vi "Struct PLC Byte Stream to G Object.vi"(8 "error in (no error)":errorcluster, 9 "[Sub-Item Type Information]":T1[](array[typedef]), 10 "Byte Stream":u8[](array[numeric]), 11 "TwinCAT ADS in":refnum<class "TwinCAT ADS.lvclass">) -> (0 "error out":errorcluster, 2 "Value":variant, 3 "TwinCAT ADS out":refnum<class "TwinCAT ADS.lvclass">)   [LabVIEW 2018, in "TwinCAT ADS.lvclass"]
uses:
  TwinCAT ADS.lvclass
  Controls/PLC Sub-Item Type Descriptor.ctl
  Controls/PLC Type.ctl
  Controls/PLC Array Type Descriptor.ctl
  Standard PLC Byte Stream to G Object.vi/9a8c356b-cf55-4838-9201-0532b80217b2.vi
  Standard PLC Byte Stream to G Object.vi/06482052-d1f9-4f29-aca9-908031c6a69f.vi
  Standard PLC Byte Stream to G Object.vi/b9242781-96b0-446e-9150-452b1084ed54.vi
  Standard PLC Byte Stream to G Object.vi/5fbe6976-0b86-40a2-b7b6-3748894f0071.vi
  Standard PLC Byte Stream to G Object.vi/c4de1741-fffd-4fed-ba25-d7b4acbf0555.vi
  Standard PLC Byte Stream to G Object.vi/20356124-05d2-4a04-a5d1-e69adc4c58c2.vi
  Standard PLC Byte Stream to G Object.vi/67ddb754-0fbe-43d9-9e61-34d6659124ef.vi
  Standard PLC Byte Stream to G Object.vi/e3d41cb3-d20e-45e9-8252-e41884a8f4d0.vi
  Standard PLC Byte Stream to G Object.vi/46ba2a54-cc07-4222-9a0e-bd972edfcef0.vi
  Standard PLC Byte Stream to G Object.vi/6b416cf7-30dc-48a3-9278-9d800f443678.vi
  Standard PLC Byte Stream to G Object.vi/5857d013-9824-4299-a2d7-53efdc0d26c5.vi
  Standard PLC Byte Stream to G Object.vi/006b0e7e-7e80-41f3-be4e-1f3da8479fae.vi
  Standard PLC Byte Stream to G Object.vi/28d9c90b-5f2a-4c58-95e2-5fc46303b0fd.vi
  Standard PLC Byte Stream to G Object.vi/99b7bc4a-962e-4818-aa5d-444f23f83b11.vi
  Standard PLC Byte Stream to G Object.vi/8b7c42c8-9170-4542-8f35-15cbeddc22cb.vi
  Standard PLC Byte Stream to G Object.vi/65a091fa-0bd2-4a35-ae2b-3fa5e90d1994.vi
  Standard PLC Byte Stream to G Object.vi/4b7d3a7d-7f1b-46f0-9357-48cb72148c56.vi
  Standard PLC Byte Stream to G Object.vi/b431183c-2ad5-4c6d-9bfa-a53b18913682.vi
  Standard PLC Byte Stream to G Object.vi/30c6c28a-53c3-4e33-80b1-b22f521e1f67.vi
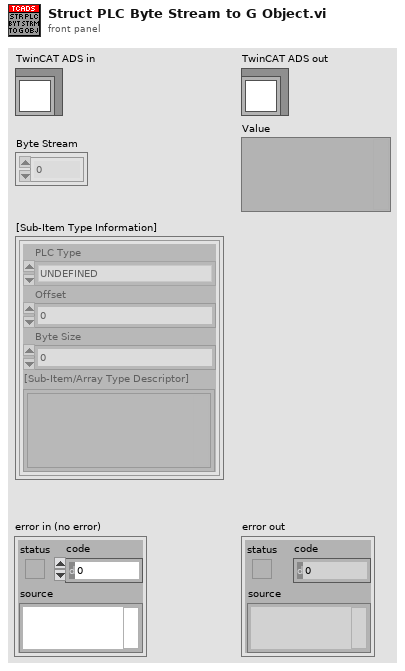
[diagram p1: front panel]
types:
  T1 = typedef "TwinCAT ADS.lvclass/PLC Sub-Item Type Descriptor.ctl" = cluster{"PLC Type":T2, "Offset":i32, "Byte Size":i32, "[Sub-Item/Array Type Descriptor]":variant[]}
  T2 = typedef "TwinCAT ADS.lvclass/PLC Type.ctl" = enum16{"UNDEFINED", "INT", "DINT", "REAL", "LREAL", "SINT", "BYTE", "UINT", "UDINT", "LINT", "ULINT", "STRING", "WSTRING", "BOOL", "TIME", "LTIME", "DATE", "DT", "TOD", "ARRAY", "JAGGED ARRAY", "STRUCT", "FUNCTION BLOCK", "POINTER", "USER DEFINED"}
  T3 = typedef "TwinCAT ADS.lvclass/PLC Array Type Descriptor.ctl" = cluster{"Fundamental PLC Type":T2, "Fundamental Type Byte Size":i32, "Item Count":i32, "Dimension Lengths":i32[], "Sub-Item Type Descriptor":variant}
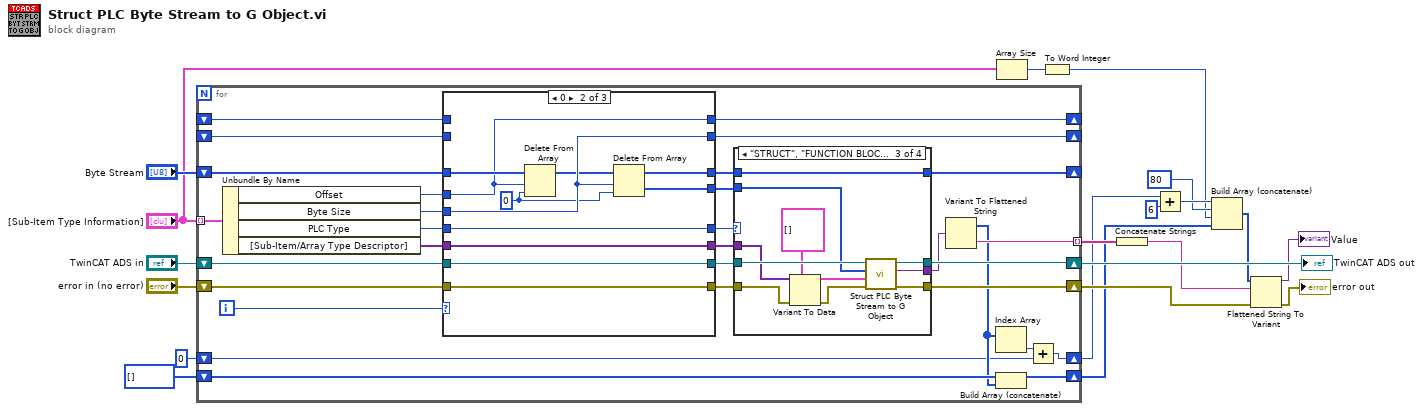
[diagram p0: block diagram]
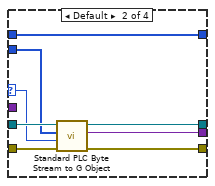
[diagram p3: hidden frame]
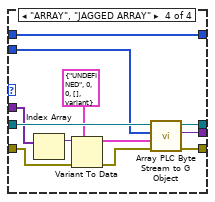
[diagram p4: hidden frame]
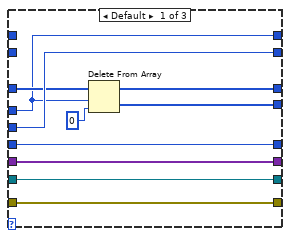
[diagram p5: hidden frame]
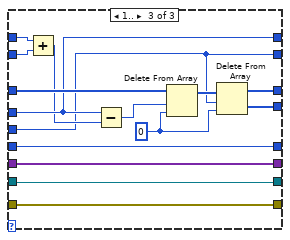
[diagram p6: hidden frame]
diagram:
  n1 = for {
    shift-right: [w46] -> _
    shift-left: "Byte Stream" -> [w38]
    shift-right: [w39] -> w9
    shift-left: "TwinCAT ADS in" -> [w50]
    shift-right: [w42] -> _
    shift-left: _ -> [w40]
    shift-right: [w43] -> _
    shift-left: _ -> [w41]
    tunnel: "[Sub-Item Type Information]" -> [w35] mode=indexing
    shift-right: [w29] -> w10
    shift-left: "error in (no error)" -> [w32]
    tunnel: [w27] -> w17 mode=indexing
    shift-right: [w25] -> w3
    shift-left: i16[] [] ("type string") -> [w26]
    shift-right: [w22] -> w1
    shift-left: i16 0 -> [w21]
    i -> [w36]
    n2 = Unbundle By Name(w35) -> ("Offset"=w34:i32, "Byte Size"=w33:i32, "PLC Type"=w30:T2, "[Sub-Item/Array Type Descriptor]"=w31:variant[])
    n3 = case shown="0" w36 {
      tunnel: w32 -> [w93 w105 w120]
      tunnel: w31 -> [w92 w103 w118]
      tunnel: w30 -> [w94 w104 w119]
      tunnel: w34 -> [w87 w97 w116]
      tunnel: w33 -> [w91 w100 w107]
      tunnel: w50 -> [w95 w106 w121]
      tunnel: w38 -> [w89 w99 w117]
      tunnel: [w95 w106 w121] -> w49
      tunnel: [w93 w105 w120] -> w48
      tunnel: [w88 w102 w115] -> w47
      tunnel: [w86 w101 w114] -> w37
      tunnel: [w94 w104 w119] -> w45
      tunnel: [w92 w103 w118] -> w44
      tunnel: [w91 w100 w107] -> w42
      tunnel: [w87 w97 w116] -> w43
      tunnel: w41 -> [_ _ w111]
      tunnel: w40 -> [_ _ w110]
      frame Default {
        n4 = Delete From Array(array=w89, length=w87, index=0) -> (deleted portion=w86:u8[], array with subset deleted=w88:u8[])
      }
      frame 0 {
        w96 = 0 ("index")
        n5 = Delete From Array(array=w99, length=w97, index=w96) -> (array with subset deleted=w98:u8[])  [unwired: 1 out]
        n6 = Delete From Array(array=w98, length=w100, index=w96) -> (deleted portion=w101:u8[], array with subset deleted=w102:u8[])
      }
      frame 1.. {
        w112 = 0 ("index")
        n7 = Add(x=w111, y=w110) -> (x+y=w109:i32)
        n8 = Subtract(x=w116, y=w109) -> (x-y=w108:i32)
        n9 = Delete From Array(array=w117, length=w108, index=w112) -> (array with subset deleted=w113:u8[])  [unwired: 1 out]
        n10 = Delete From Array(array=w113, length=w107, index=w112) -> (deleted portion=w114:u8[], array with subset deleted=w115:u8[])
      }
    }
    n11 = case shown="\"STRUCT\", \"FUNCTION BLOCK\"" w45 {
      selector: w45 -> [_ w58 _ _]
      tunnel: w49 -> [w53 w62 w72 w85]
      tunnel: w48 -> [w52 w61 w67 w78]
      tunnel: w47 -> [w54 w59 w73 w84]
      tunnel: w37 -> [w51 w60 w71 w80]
      tunnel: [w54 w59 w73 w84] -> w46
      tunnel: [w53 w57 w70 w82] -> w39
      tunnel: [w52 w56 w68 w83] -> w29
      tunnel: [w51 w55 w69 w81] -> w28
      tunnel: w44 -> [_ _ w66 w79]
      frame "UNDEFINED" {
      }
      frame Default {
        n12 = call "Standard PLC Byte Stream to G Object.vi"("error in (no error)"=w61, "PLC Type"=w58, "Byte Stream"=w60, "TwinCAT ADS in"=w62) -> ("error out"=w56:errorcluster, "Value"=w55:variant, "TwinCAT ADS out"=w57:refnum<class "TwinCAT ADS.lvclass">)  [unwired: 5 in]
      }
      frame "STRUCT", "FUNCTION BLOCK" {
        n13 = Variant To Data(error in=w67, type=T1[] [] ("[Sub-Item Type Information]"), Variant=w66) -> (data=w63:T1[], error out=w64:errorcluster)
        n14 = call "Struct PLC Byte Stream to G Object.vi"("error in (no error)"=w64, "[Sub-Item Type Information]"=w63, "Byte Stream"=w71, "TwinCAT ADS in"=w72) -> ("error out"=w68:errorcluster, "Value"=w69:variant, "TwinCAT ADS out"=w70:refnum<class "TwinCAT ADS.lvclass">)  [unwired: 5 in]
      }
      frame "ARRAY", "JAGGED ARRAY" {
        n15 = Index Array(array=w79) -> (element=w77:variant)  [unwired: 1 in]
        n16 = Variant To Data(error in=w78, type=T3 {"Fundamental PLC Type"=enum."UNDEFINED", "Fundamental Type Byte Size"=0, "Item Count"=0, "Dimension Lengths"=[], "Sub-Item Type Descriptor"=variant} ("Array Information"), Variant=w77) -> (data=w75:T3, error out=w76:errorcluster)
        n17 = call "Array PLC Byte Stream to G Object.vi"("error in (no error)"=w76, "Array Type Descriptor"=w75, "Byte Stream"=w80, "TwinCAT ADS in"=w85) -> ("error out"=w83:errorcluster, "Value"=w81:variant, "TwinCAT ADS out"=w82:refnum<class "TwinCAT ADS.lvclass">)  [unwired: 5 in]
      }
    }
    n18 = Variant To Flattened String(Variant=w28) -> (data string=w27:string, 1:w24:i16[])
    n19 = Index Array(array=w24) -> (element=w23:i16)  [unwired: 1 in]
    n20 = Build Array (concatenate)(w26, w24) -> (w25:i16[])
    n21 = Add(x=w23, y=w21) -> (x+y=w22:i16)
  }
  "TwinCAT ADS out" <- w9
  n22 = Array Size(array="[Sub-Item Type Information]") -> (size(s)=w15:i32)
  n23 = To Word Integer(number=w15) -> (16bit integer=w11:i16)
  n24 = Concatenate Strings(w17) -> (w8:string)
  n25 = Add(x=w1, y=i16 6) -> (x+y=w13:i16)
  n26 = Build Array (concatenate)(w13, i16 80, w11, w3) -> (w7:i16[])
  n27 = Flattened String To Variant(4:w10, 6:w8, 7:w7) -> (0:→"error out":errorcluster, 3:→"Value":variant)
